vi "JoystickTester.vi"() -> ()   [LabVIEW 2018]
uses:
  <vilib>/Platform/TimedLoop/XDataNode/timing_clust.ctl
  <vilib>/Platform/TimedLoop/XDataNode/nitl_modes.ctl
  <vilib>/Platform/TimedLoop/XDataNode/wakeup.ctl
  <vilib>/rvi/Emulation/niFpgaSctlEmulationGetInTimedLoop.vi
  <vilib>/rvi/Emulation/niFpgaEmulationReportErrorSimple.vi
  <vilib>/rvi/Emulation/niFpgaGetClockAttributes.vi
  <vilib>/rvi/Emulation/niFpgaCriticalErrorInLSC.vi
  <vilib>/rvi/eio/common/nirviEmuTemplateMethod_errors.vi
  <vilib>/platform/TimedLoop/XDataNode/XDataNode.xnode
  <vilib>/eio/EIONode/EIONode.xnode
  <vilib>/Platform/TimedLoop/XDataNode/XDNodeRunTimeDep.lvlib
panel:
  out "Joy4_Up":bool
  out "Joy4_Down":bool
  out "Joy4_Left":bool
  out "Joy4_Right":bool
  out "Joy4_Button":bool
  out "Joy3_Up":bool
  out "Joy3_Down":bool
  out "Joy3_Left":bool
  out "Joy3_Right":bool
  out "Joy3_Button":bool
  out "Joy2_Up":bool
  out "Joy2_Down":bool
  out "Joy2_Left":bool
  out "Joy2_Right":bool
  out "Joy2_Button":bool
  out "Joy1_Button":bool
  out "Joy1_Right":bool
  out "Joy1_Left":bool
  out "Joy1_Down":bool
  out "Joy1_Up":bool
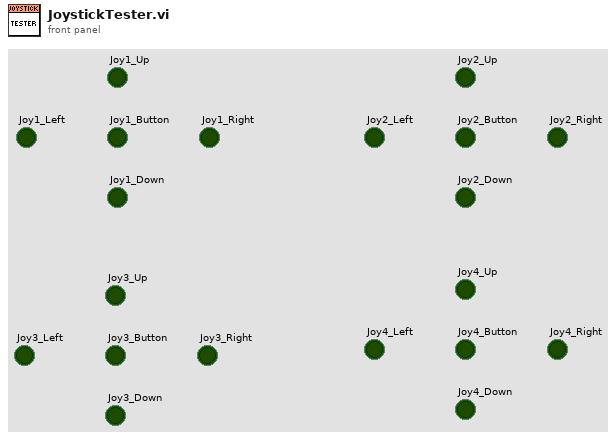
[diagram p1: front panel]
types:
  T1 = typedef "XDNodeRunTimeDep.lvlib/timing_clust.ctl" = cluster{"Expected End [f-1]":u64, "Actual End [f-1]":u64, "Finished Late? [f-1]":bool, "Expected End [i-1]":u64, "Actual End [i-1]":u64, "Finished Late? [i-1]":bool, "Expected Start [i]":u64, "Actual Start [i]":u64, "Expected Start [f]":u64, "Actual Start [f]":u64, "Source Name":string, "Structure Name":string, "Period":i64, "Deadline":i64, "Offset":i64, "Start":i64, "Priority":i32, "Timeout":i32, "Mode":T2, "Wakeup Reason":T3, "Error":errorcluster, "Source Type":string, "Secondary Source Type":string, "Global End Time":u64, "Global Start Time":u64, "Frame Duration":u64, "Iteration Duration":u64, "Assigned CPU":i32, "I/O Scan Engine Mode":u32}
  T2 = typedef "XDNodeRunTimeDep.lvlib/nitl_modes.ctl" = enum32{"No Change", "Process missed periods, maintain original phase", "Discard missed periods, maintain original phase", "Process missed periods, ignore original phase", "Discard missed periods, ignore original phase"}
  T3 = typedef "XDNodeRunTimeDep.lvlib/wakeup.ctl" = enum32{"Normal", "Aborted", "Asynchronous wakeup", "Timing source error", "Timed loop error", "Timeout"}
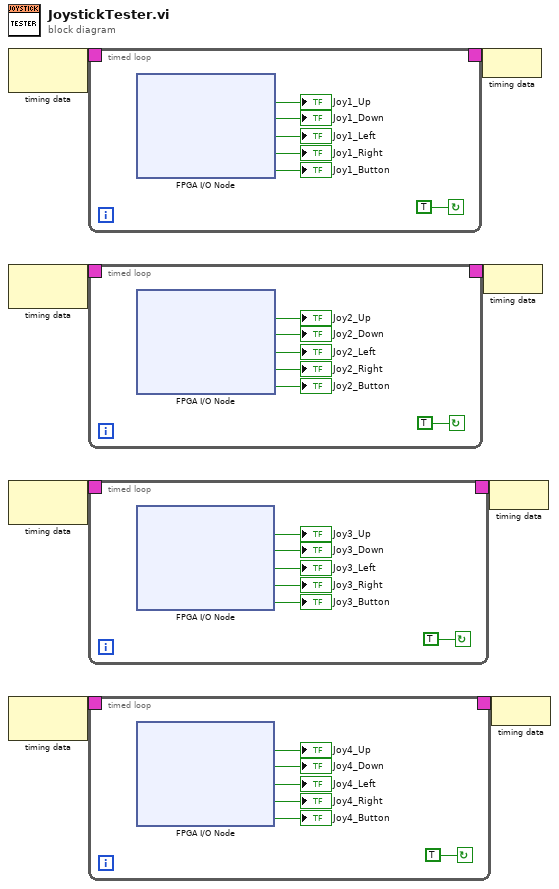
[diagram p0: block diagram]
diagram:
  n1 = node-c288() -> (w8:T1)  [unwired: 1 in]
  n2 = node-c288() -> (w6:T1)  [unwired: 1 in]
  n3 = node-c288() -> (w4:T1)  [unwired: 1 in]
  n4 = node-c288() -> (w2:T1)  [unwired: 1 in]
  n5 = timed-loop {
    timing: w8 -> [_]
    timing-out: [_] -> w7
    stop <- TRUE continue-if-true
    n6 = xnode "FPGA I/O Node"() -> ("ConnectorA/DIO0"=→"Joy1_Up":bool, "ConnectorA/DIO1"=→"Joy1_Down":bool, "ConnectorA/DIO2"=→"Joy1_Left":bool, "ConnectorA/DIO3"=→"Joy1_Right":bool, "ConnectorA/DIO4"=→"Joy1_Button":bool)  [unwired: 5 in, 5 out]
  }
  n7 = timed-loop {
    timing: w6 -> [_]
    timing-out: [_] -> w5
    stop <- TRUE continue-if-true
    n8 = xnode "FPGA I/O Node"() -> ("ConnectorA/DIO5"=→"Joy2_Up":bool, "ConnectorA/DIO6"=→"Joy2_Down":bool, "ConnectorA/DIO7"=→"Joy2_Left":bool, "ConnectorA/DIO8"=→"Joy2_Right":bool, "ConnectorA/DIO9"=→"Joy2_Button":bool)  [unwired: 5 in, 5 out]
  }
  n9 = timed-loop {
    timing: w4 -> [_]
    timing-out: [_] -> w3
    stop <- TRUE continue-if-true
    n10 = xnode "FPGA I/O Node"() -> ("ConnectorB/DIO0"=→"Joy3_Up":bool, "ConnectorB/DIO1"=→"Joy3_Down":bool, "ConnectorB/DIO2"=→"Joy3_Left":bool, "ConnectorB/DIO3"=→"Joy3_Right":bool, "ConnectorB/DIO4"=→"Joy3_Button":bool)  [unwired: 5 in, 5 out]
  }
  n11 = timed-loop {
    timing: w2 -> [_]
    timing-out: [_] -> w1
    stop <- TRUE continue-if-true
    n12 = xnode "FPGA I/O Node"() -> ("ConnectorB/DIO5"=→"Joy4_Up":bool, "ConnectorB/DIO6"=→"Joy4_Down":bool, "ConnectorB/DIO7"=→"Joy4_Left":bool, "ConnectorB/DIO8"=→"Joy4_Right":bool, "ConnectorB/DIO9"=→"Joy4_Button":bool)  [unwired: 5 in, 5 out]
  }
  n13 = node-c288(w7) -> ()
  n14 = node-c288(w5) -> ()
  n15 = node-c288(w3) -> ()
  n16 = node-c288(w1) -> ()
